vi "Gaussian Modulated Sine Pattern.vi"(5 "attenuation (dB)":dbl=6.0, 6 "normalized bandwidth":dbl=0.15, 7 "center frequency (Hz)":dbl=1.0, 8 "delta t (s)":dbl=0.1, 9 "delay (s)":dbl, 10 "amplitude":dbl=1.0, 11 "samples":i32=128) -> (0 "error":i32, 3 "Gauss-Mod Sine Pattern":dbl[](array[numeric]))   [LabVIEW 2017, in "NI_AALBase.lvlib"]
doc: "Generates an array that contains a Gaussian-modulated sinusoidal pattern."
uses:
  <vilib>/Analysis/NI_AALBase.lvlib
panel:
  # "Gaussian Modulated Sine Pattern"
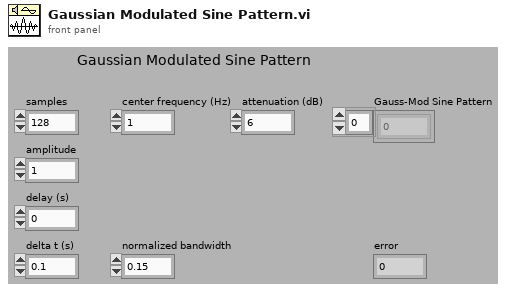
[diagram p1: front panel]
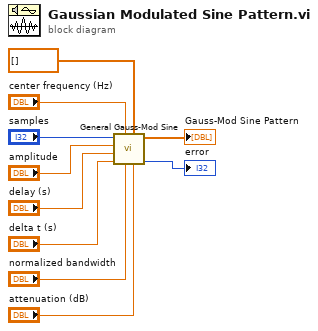
[diagram p0: block diagram]
diagram:
  n1 = call <vilib>:"General Gauss-Mod Sine.vi"("attenuation"="attenuation (dB)", "X"=dbl[] [] ("x"), "bandwidth"="normalized bandwidth", "center frequency"="center frequency (Hz)", "delta t"="delta t (s)", "delay"="delay (s)", "amplitude"="amplitude", "samples"="samples") -> ("error"=→"error":i32, "Gauss-Mod Sine Pattern"=→"Gauss-Mod Sine Pattern":dbl[])  [unwired: 2 in]
